vi "TESTE.vi"() -> ()   [LabVIEW 2018]
panel:
  out "error out 2":errorcluster
  out "return value 2":string
  out "return value":string
  out "error out":errorcluster
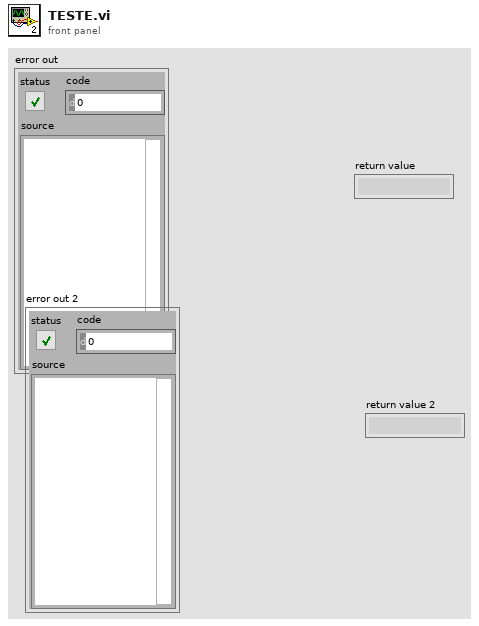
[diagram p1: front panel]
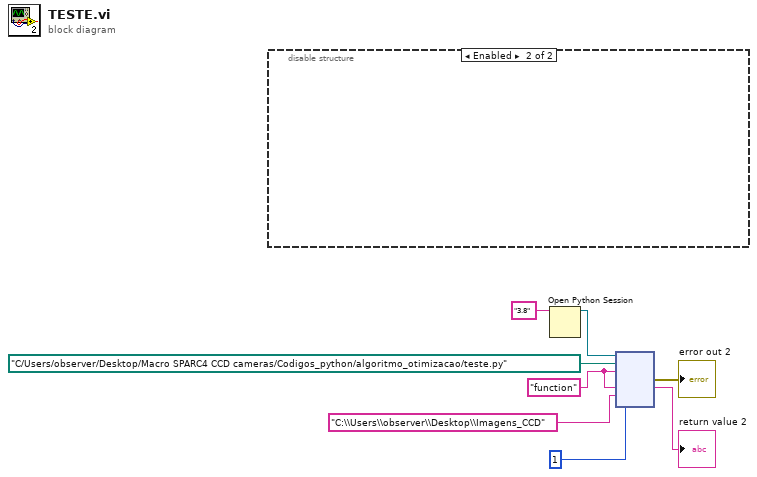
[diagram p0: block diagram]
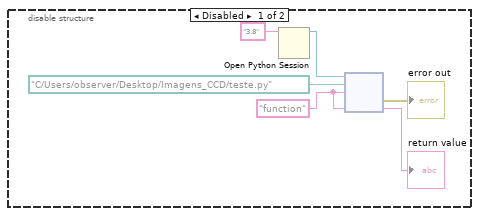
[diagram p2: hidden frame]
diagram:
  w8 = "function" ("function name")
  n1 = disable-structure shown="Enabled" {
    frame Disabled {
      w9 = "function" ("function name")
      n2 = Open Python Session(python version="3.8" ("Python version")) -> (session out=w13:refnum<k35>)  [unwired: 2 in, 1 out]
      n3 = node(w13, path "C:/Users/observer/Desktop/Imagens_CCD/teste.py" ("module path"), w9, w9) -> (→"error out":errorcluster, →"return value":string)  [unwired: 1 in, 3 out]
    }
    frame Enabled {
    }
  }
  n4 = Open Python Session(python version="3.8" ("Python version")) -> (session out=w4:refnum<k35>)  [unwired: 2 in, 1 out]
  n5 = node(w4, path "C:/Users/observer/Desktop/Macro SPARC4 CCD cameras/Codigos_python/algoritmo_otimizacao/teste.py" ("module path"), w8, w8, "C:\\Users\\observer\\Desktop\\Imagens_CCD" ("function name"), 1) -> (→"error out 2":errorcluster, →"return value 2":string)  [unwired: 3 in, 3 out]
